vi "Error_Trans.vi"(5 "Remove code":bool, 7 "Remove ===":bool=TRUE, 8 "Error In":errorcluster, 9 "VAR":variant, 10 "Add_s%":bool, 11 "noCallChain[T]":bool=TRUE) -> (0 "Error Out":errorcluster, 1 "Message":string)   [LabVIEW 2020, in "Main.lvlib"]
doc: "Read error ring of ILL Error codes and generate a string for the log."
uses:
  Main.lvlib
  <vilib>/Utility/error.llb/DialogType.ctl
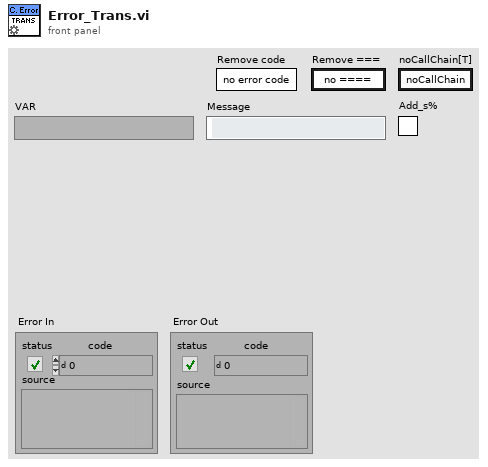
[diagram p1: front panel]
types:
  T1 = typedef "DialogType.ctl" = u16
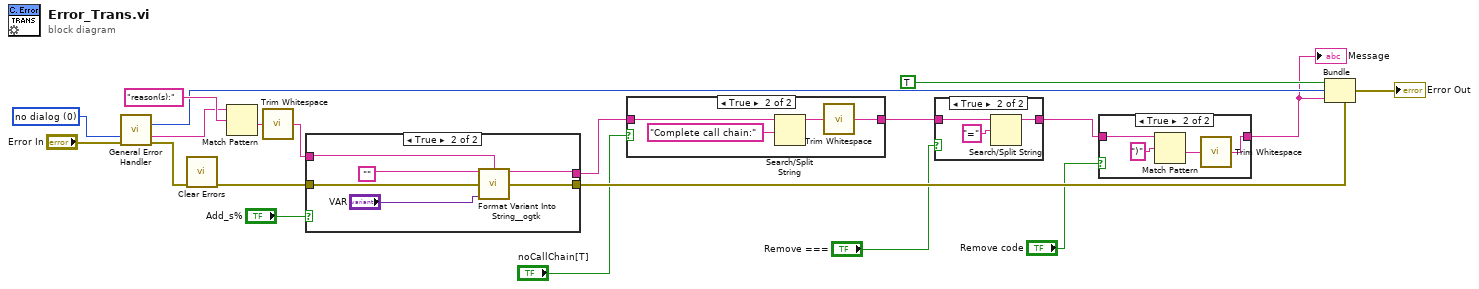
[diagram p0: block diagram]
diagram:
  w20 = T1 0 items=["no dialog", "OK message", "continue or stop message", "OK message + warnings", "continue/stop + warnings"] ("type of dialog (OK msg:1)")
  n1 = call <vilib>:"General Error Handler.vi"("type of dialog (OK msg:1)"=w20, "error in (no error)"="Error In") -> ("code out"=w16:i32, "message"=w18:string, "error out"=w11:errorcluster)  [unwired: 9 in, 2 out]
  n2 = call <vilib>:"Clear Errors.vi"("error in (no error)"=w11) -> ("error out"=w13:errorcluster)  [unwired: 5 in, 1 out]
  n3 = Match Pattern(string=w18, regular expression="reason(s):") -> (after substring=w17:string)  [unwired: 1 in, 3 out]
  n4 = call <vilib>:"Trim Whitespace.vi"("string"=w17) -> ("trimmed string"=w14:string)  [unwired: 1 in]
  n5 = case shown="True" "Add_s%" {
    tunnel: w14 -> [w22 w24]
    tunnel: [w22 w23] -> w9
    tunnel: w13 -> [w21 w28]
    tunnel: [w21 w27] -> w12
    frame False {
    }
    frame True {
      n6 = call <userlib>:"Format Variant Into String__ogtk.vi"("Input String"="", "Format String"=w24, "error in (no error)"=w28, "Variant"="VAR") -> ("Output String"=w23:string, "error out"=w27:errorcluster)  [unwired: 10 in]
    }
  }
  n7 = case shown="True" "noCallChain[T]" {
    tunnel: w9 -> [w29 w33]
    tunnel: [w29 w30] -> w7
    frame False {
    }
    frame True {
      n8 = Search/Split String(string=w33, search string/char (-)="Complete call chain:" ("regular expression")) -> (substring before match=w31:string)  [unwired: 1 in, 2 out]
      n9 = call <vilib>:"Trim Whitespace.vi"("string"=w31) -> ("trimmed string"=w30:string)  [unwired: 1 in]
    }
  }
  n10 = case shown="True" "Remove ===" {
    tunnel: w7 -> [w34 w37]
    tunnel: [w34 w35] -> w5
    frame False {
    }
    frame True {
      n11 = Search/Split String(string=w37, search string/char (-)="=") -> (substring before match=w35:string)  [unwired: 1 in, 2 out]
    }
  }
  n12 = case shown="True" "Remove code" {
    tunnel: w5 -> [w38 w42]
    tunnel: [w38 w39] -> w4
    frame False {
    }
    frame True {
      n13 = Match Pattern(string=w42, regular expression=")" ("search string/char (-)")) -> (after substring=w40:string)  [unwired: 1 in, 3 out]
      n14 = call <vilib>:"Trim Whitespace.vi"("string"=w40) -> ("trimmed string"=w39:string)  [unwired: 1 in]
    }
  }
  "Message" <- w4
  n15 = Bundle(cluster=w12, "status"=TRUE, "code"=w16, "source"=w4) -> (→"Error Out":errorcluster)
